vi "P9374A NA port source enable.vi"(7 "Enable":bool, 8 "error in (no error)":errorcluster {"code" format="%.0x"}, 10 "Port":string(combo)="2", 11 "instrument handle in":refnum<k15> caption="instrument handle out") -> (0 "error out":errorcluster {"code" format="%.0x"}, 3 "instrument handle out":refnum<k15>)   [LabVIEW 2021]
uses:
  <instrlib>/Agilent NA/Agilent NA.lvlib
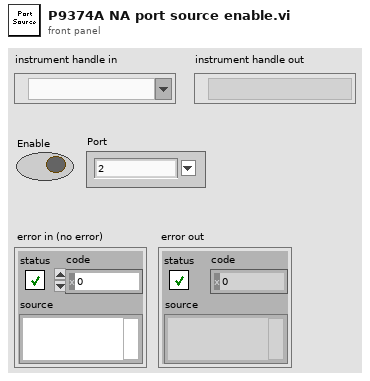
[diagram p1: front panel]
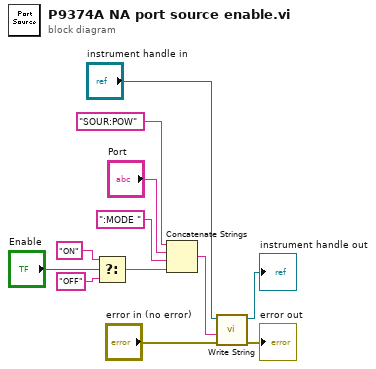
[diagram p0: block diagram]
diagram:
  n1 = Select(t="ON", s="Enable", f="OFF") -> (s? t:f=w5:string)
  n2 = Concatenate Strings("SOUR:POW" ("string"), "Port", ":MODE " ("string"), w5) -> (w4:string)
  n3 = call <instrlib>:"Write String.vi"("error in (no error)"="error in (no error)", "Command"=w4, "instrument handle"="instrument handle in") -> ("error out"=→"error out":errorcluster, "instrument handle out"=→"instrument handle out":refnum<k15>)  [unwired: 7 in]
